vi "LocalQueue_Test Disconnected by Peer.vi"(8 "error in (no error)":errorcluster) -> (0 "error out":errorcluster)   [LabVIEW 2013]
uses:
  <vilib>/addons/_JKI Toolkits/Caraya/classes/Assert/Assert Not Error.vi
  <vilib>/addons/_JKI Toolkits/Caraya/classes/Assert/Assert Equal Value_Variant.vi
  <vilib>/addons/_JKI Toolkits/Caraya/classes/Test/Test.lvclass
  <vilib>/addons/_JKI Toolkits/Caraya/classes/Assert/Assert.lvclass
  <vilib>/LabVIEW Open Source Project/MQTT Connection/MQTT_Connection/Connection/Connection.lvclass
  source/MQTT_LocalQueue/Connection/LocalQueueConnection.lvclass
panel:
  out "connected":bool
  out "server connected":bool
  out "client connected":bool
  out "Comm OK":bool
  out "value":dbl
  out "Bytes":u8[](array[numeric]) format="%08b"
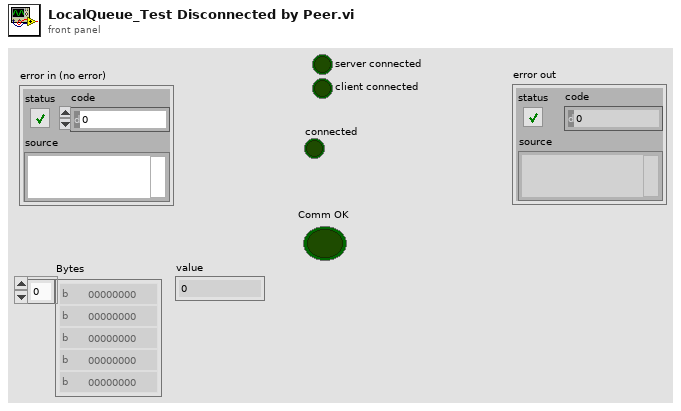
[diagram p1: front panel]
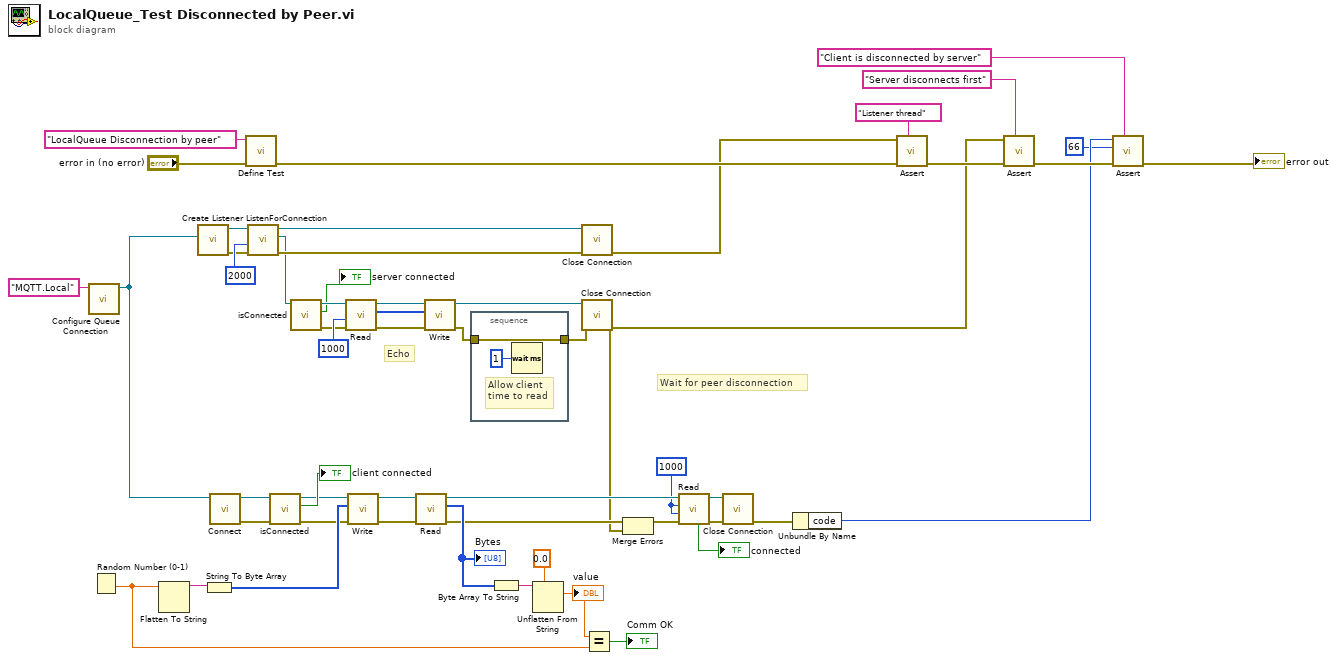
[diagram p0: block diagram]
diagram:
  w12 = 1000 ("bytes to read (100)")
  # "Wait for peer disconnection"
  # "Echo"
  n1 = call "Configure Queue Connection.vi"("Queue Name"="MQTT.Local") -> ("LocalQueueConnection"=w1:refnum<class "LocalQueueConnection.lvclass">)  [unwired: 9 in, 1 out]
  n2 = Random Number (0-1)() -> (number: 0 to 1=w27:dbl)
  n3 = Flatten To String(anything=w27) -> (data string=w34:string)  [unwired: 3 in, 2 out]
  n4 = call <vilib>:"Create Listener.vi"("Connection Configuration"=w1) -> ("error out"=w42:errorcluster, "Listener"=w45:refnum<class "Connection.lvclass">)  [unwired: 9 in]
  n5 = String To Byte Array(string=w34) -> (unsigned byte array=w33:u8[])
  n6 = call <vilib>:"Connect.vi"("Connection in"=w1) -> ("error out"=w22:errorcluster, "Connection out"=w20:refnum<class "LocalQueueConnection.lvclass">)  [unwired: 9 in]
  n7 = call <vilib>:"Define Test.vi"("error in (no error)"="error in (no error)", "Label (VI Title)"="LocalQueue Disconnection by peer") -> ("error out"=w53:errorcluster)  [unwired: 9 in]
  n8 = call <vilib>:"ListenForConnection.vi"("error in (no error)"=w42, "timeout (2000 ms)"=2000 ("bytes to read (100)"), "Listener"=w45) -> ("error out"=w29:errorcluster, "Connection"=w18:refnum<class "Connection.lvclass">, "Listener out"=w43:refnum<class "Connection.lvclass">)  [unwired: 5 in, 1 out]
  n9 = call <vilib>:"isConnected.vi"("error in (no error)"=w22, "Connection in"=w20) -> ("error out"=w21:errorcluster, "connected"=→"client connected":bool, "Connection out"=w19:refnum<class "LocalQueueConnection.lvclass">)  [unwired: 7 in]
  n10 = call <vilib>:"isConnected.vi"("Connection in"=w18) -> ("error out"=w16:errorcluster, "connected"=→"server connected":bool, "Connection out"=w17:refnum<class "Connection.lvclass">)  [unwired: 8 in]
  n11 = call <vilib>:"Read.vi"("error in (no error)"=w16, "timeout (2000 ms)"=1000 ("bytes to read (100)"), "TCPConnection in"=w17) -> ("error out"=w37:errorcluster, "Bytes"=w39:u8[], "TCPConnection out"=w40:refnum<class "Connection.lvclass">)  [unwired: 4 in, 2 out]
  n12 = call <vilib>:"Write.vi"("error in (no error)"=w21, "Bytes"=w33, "Connection in"=w19) -> ("error out"=w36:errorcluster, "Connection"=w38:refnum<class "LocalQueueConnection.lvclass">)  [unwired: 7 in]
  n13 = call <vilib>:"Read.vi"("error in (no error)"=w36, "TCPConnection in"=w38) -> ("error out"=w8:errorcluster, "Bytes"=w32:u8[], "TCPConnection out"=w14:refnum<class "LocalQueueConnection.lvclass">)  [unwired: 5 in, 2 out]
  "Bytes" <- w32
  n14 = call <vilib>:"Write.vi"("error in (no error)"=w37, "Bytes"=w39, "Connection in"=w40) -> ("error out"=w25:errorcluster, "Connection"=w35:refnum<class "Connection.lvclass">)  [unwired: 7 in]
  n15 = stacked-sequence {
    tunnel: w25 -> [w55]
    tunnel: [w55] -> w24
    frame #0 {
      # "Allow client\ntime to read"
      n16 = Wait (ms)(milliseconds to wait=u32 1) -> ()  [unwired: 1 out]
    }
  }
  n17 = Byte Array To String(unsigned byte array=w32) -> (string=w31:string)
  n18 = Unflatten From String(type=0.0, binary string=w31) -> (value=w28:dbl)  [unwired: 3 in, 2 out]
  "value" <- w28
  n19 = call <vilib>:"Close Connection.vi"("error in (no error)"=w29, "Connection in"=w43) -> ("error out"=w11:errorcluster)  [unwired: 8 in, 1 out]
  n20 = call <vilib>:"Close Connection.vi"("error in (no error)"=w24, "Connection in"=w35) -> ("error out"=w7:errorcluster)  [unwired: 8 in, 1 out]
  n21 = Equal?(x=w28, y=w27) -> (x = y?=→"Comm OK":bool)
  n22 = Merge Errors(w8, w7) -> (w6:errorcluster)
  n23 = call <vilib>:"Read.vi"("error in (no error)"=w6, "timeout (2000 ms)"=w12, "bytes to read (100)"=w12, "TCPConnection in"=w14) -> ("error out"=w9:errorcluster, "TCPConnection out"=w13:refnum<class "LocalQueueConnection.lvclass">, "connected"=→"connected":bool)  [unwired: 3 in, 2 out]
  n24 = call <vilib>:"Close Connection.vi"("error in (no error)"=w9, "Connection in"=w13) -> ("error out"=w10:errorcluster)  [unwired: 8 in, 1 out]
  n25 = Unbundle By Name(w10) -> ("code"=w50:i32)
  n26 = call-poly <vilib>:"Assert.vi"("Label"="Listener thread" ("Label (VI Title)"), "error in (no error)"=w53, "Not Error?"=w11) -> ("error out"=w52:errorcluster)  [unwired: 8 in]
  n27 = call-poly <vilib>:"Assert.vi"("Label"="Server disconnects first" ("Label (VI Title)"), "error in (no error)"=w52, "Not Error?"=w7) -> ("error out"=w51:errorcluster)  [unwired: 8 in]
  n28 = call-poly <vilib>:"Assert.vi"("Label"="Client is disconnected by server" ("Label (VI Title)"), "error in (no error)"=w51, "Y"=66 ("code"), "X"=w50) -> ("error out"=→"error out":errorcluster)  [unwired: 7 in]
